vi "Actor Core.vi"(8 "error in":errorcluster, 11 "Study Actor in":refnum<class "Study Actor.lvclass">) -> (0 "error out":errorcluster, 3 "Actor out":refnum<class "Actor.lvclass">)   [LabVIEW 2024, in "Study Actor.lvlib" / "Study Actor.lvclass"]
doc: "The user interface for this panel.\n\n----\nPlease see the following web address for additional documentation and tutorial information:\nhttp://www.mooregoodideas.com/mgi-panel-manager/\n\nAuthor: Derek Trepanier\n\nCopyright (c) 2018, Moore Good Ideas, Inc.\n\nAll rights reserved.\n\nRedistribution and use in source and binary forms, with or without modification, are permitted provided that the following conditions are met:\n\n * Redistributions of source code must retain the above copyright notice, this list of conditions and the following disclaimer.\n * Redistributions in binary form must reproduce the above copyright notice, this list of conditions and the following disclaimer in the documentation and/or other materials provided with the distribution.\n * Neither the name of Moore Good Ideas, Inc. nor the names of its contributors may be used to endorse or promote products derived from this software without specific prior written permission.\n\nTHIS SOFTWARE IS PROVIDED BY THE COPYRIGHT HOLDERS AND CONTRIBUTORS \"AS IS\" AND ANY EXPRESS OR IMPLIED WARRANTIES, INCLUDING, BUT NOT LIMITED TO, THE IMPLIED WARRANTIES OF MERCHANTABILITY AND FITNESS FOR A PARTICULAR PURPOSE ARE DISCLAIMED. IN NO EVENT SHALL THE COPYRIGHT OWNER OR CONTRIBUTORS BE LIABLE FOR ANY DIRECT, INDIRECT, INCIDENTAL, SPECIAL, EXEMPLARY, OR CONSEQUENTIAL DAMAGES (INCLUDING, BUT NOT LIMITED TO, PROCUREMENT OF SUBSTITUTE GOODS OR SERVICES; LOSS OF USE, DATA, OR PROFITS; OR BUSINESS INTERRUPTION) HOWEVER CAUSED AND ON ANY THEORY OF LIABILITY, WHETHER IN CONTRACT, STRICT LIABILITY, OR TORT (INCLUDING NEGLIGENCE OR OTHERWISE) ARISING IN ANY WAY OUT OF THE USE OF THIS SOFTWARE, EVEN IF ADVISED OF THE POSSIBILITY OF SUCH DAMAGE."
uses:
  Study Actor.lvclass
  C:/Program Files/National Instruments/LabVIEW 2024/vi.lib/MGI/Panel Manager/Panel Actor/Panel Actor/Panel Actor.lvclass
  <vilib>/ActorFramework/Actor/Actor.lvclass
  Study Actor.lvclass/Study Actor.ctl
  <vilib>/ActorFramework/Message Enqueuer/Message Enqueuer.lvclass/Message Enqueuer.ctl
  IStudy Actor Messages/Log Target Msg/Log Target Msg.lvclass/Log Target Msg.ctl
  <vilib>/ActorFramework/Message Enqueuer/Enqueue.vi
  <vilib>/ActorFramework/Stop Msg/Stop Msg.lvclass
  C:/Program Files/National Instruments/LabVIEW 2024/vi.lib/ActorFramework/Message/Message.lvclass
  Study Actor Messages/Stop Target Actor Msg/Stop Target Actor Msg.lvclass
  IStudy Actor Messages/Log Target Msg/Log Target Msg.lvclass
  <vilib>/Utility/LVClass/Get LV Class Name.vi
  <resource>/AFDebug/Generate Trace for Message.vi
  <vilib>/ActorFramework/Message Priority Queue/Priority Enqueue.vi
  <vilib>/MGI/Panel Manager/Panel Actor/Panel Actor/Panel Actor.lvclass
  C:/Program Files/National Instruments/LabVIEW 2024/vi.lib/ActorFramework/Actor/Actor.lvclass
  D:/git/HAL/MAL/Study/Study Actor/Study Actor/Study Actor.lvclass
  D:/git/HAL/MAL/Study/Study Actor/IStudy Actor/IStudy Actor.lvclass
  C:/Program Files/National Instruments/LabVIEW 2024/vi.lib/ni/Actors/Network Endpoint Actors/Nested Endpoint Caller/Nested Endpoint Caller/Nested Endpoint Caller.lvclass
panel:
  in  "Launch Target":bool
  in  "Kill Target Button":bool
  out "Target Log":string
  out "Target Connected":bool
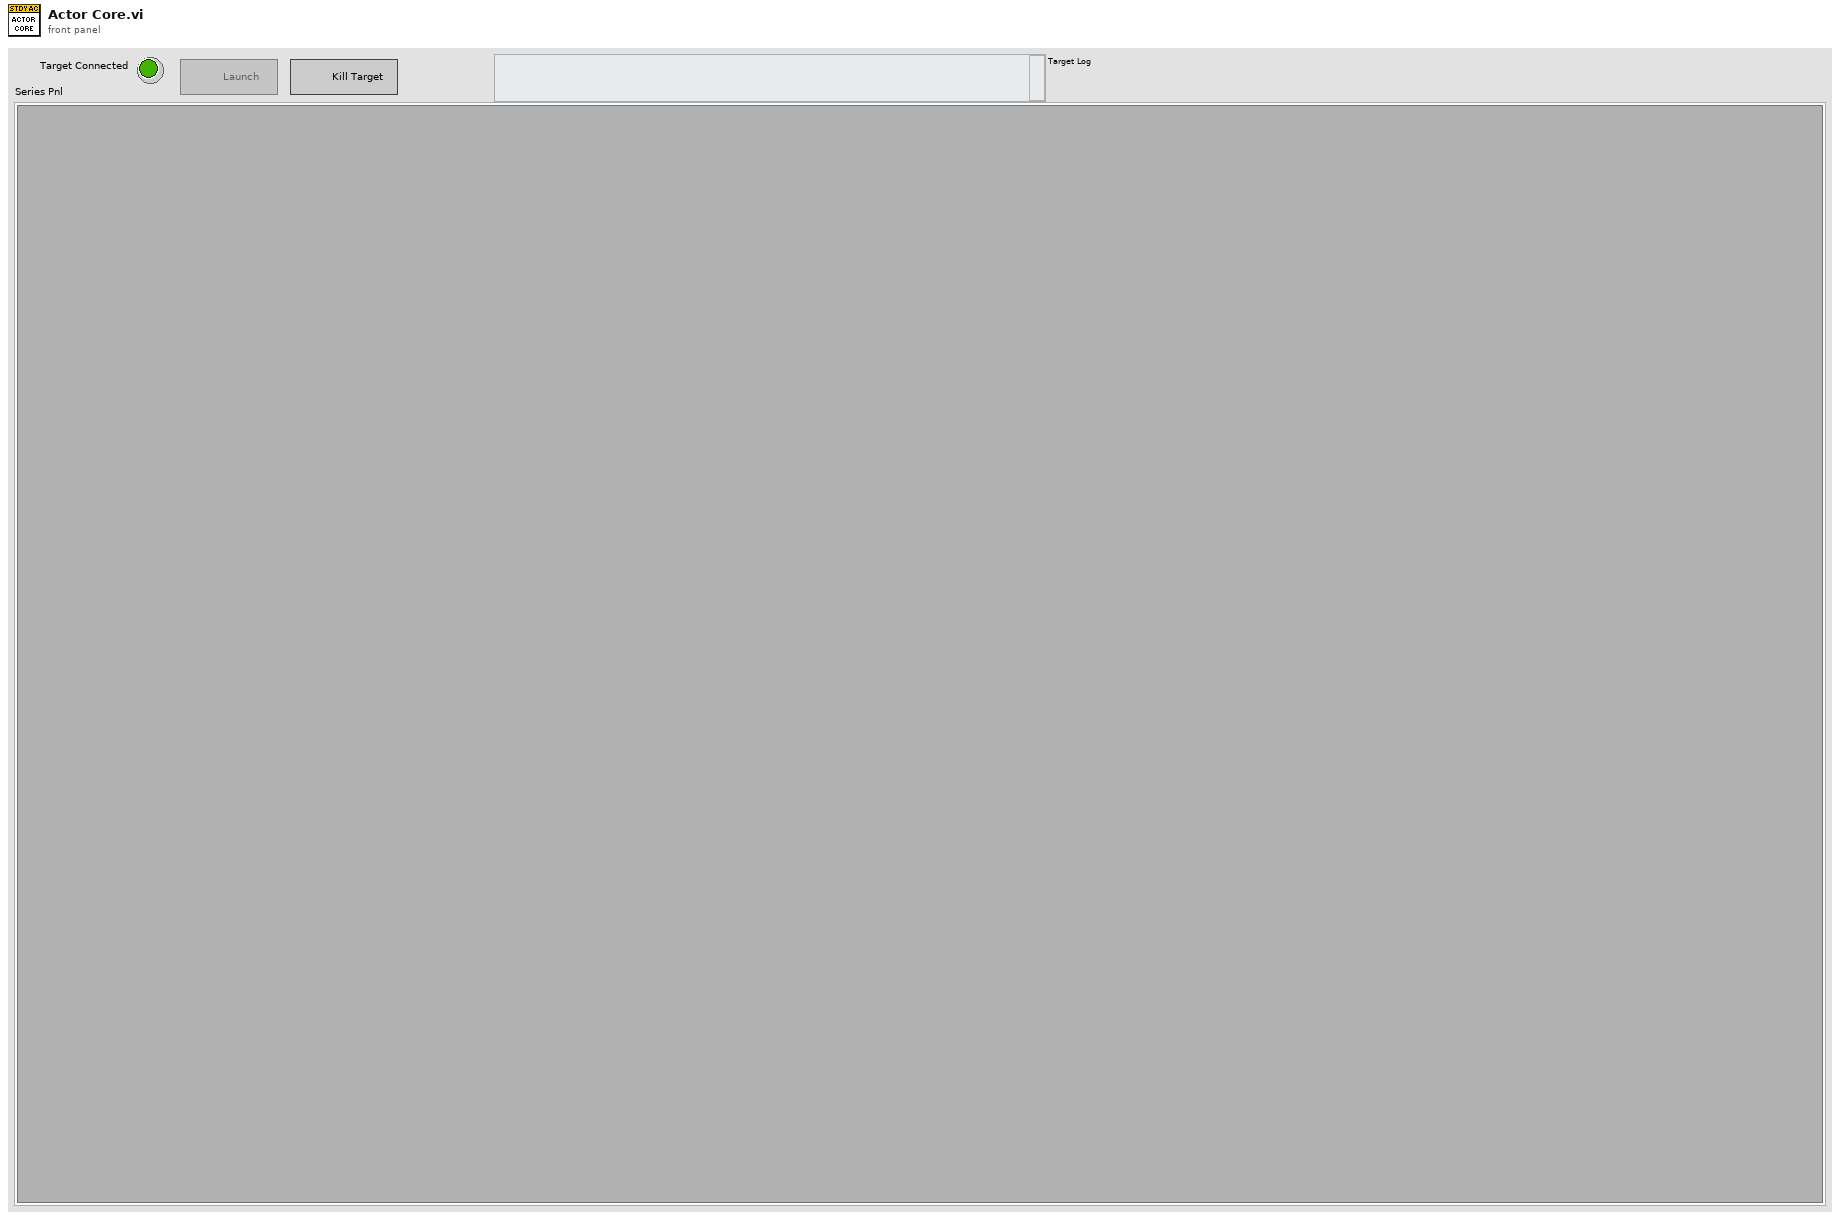
[diagram p1: front panel]
types:
  T1 = cluster{"Connected":refnum<user-event>, "Target Log Entry":refnum<user-event>}
  T2 = cluster{"Pnl Actor":refnum<event-registration>, "Event Registration Refnum":refnum<event-registration>}
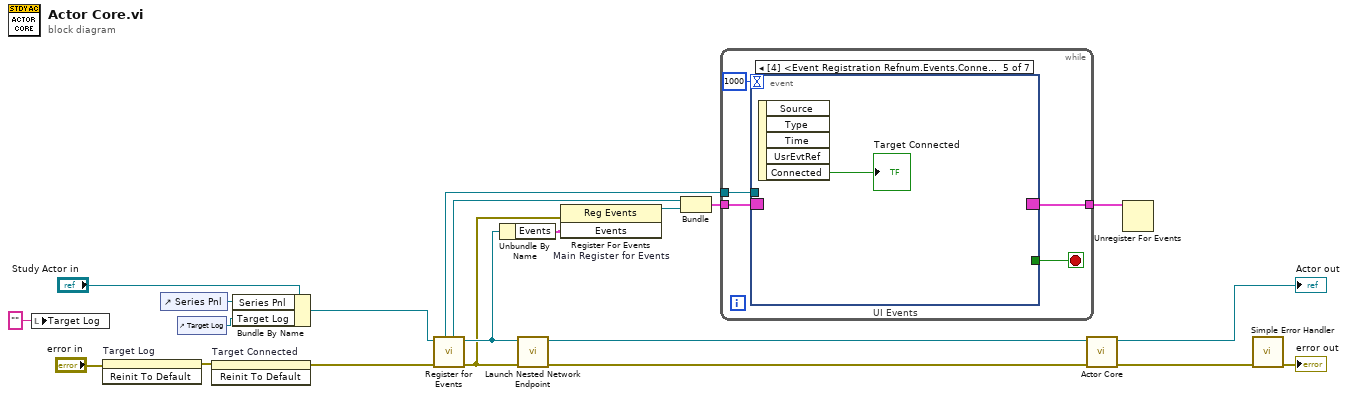
[diagram p0: block diagram]
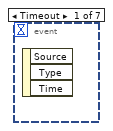
[diagram p2: hidden frame]
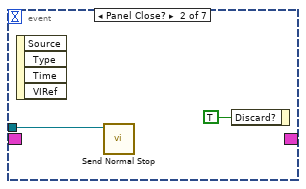
[diagram p3: hidden frame]
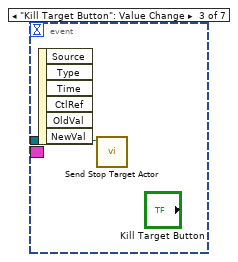
[diagram p4: hidden frame]
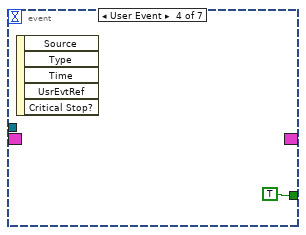
[diagram p5: hidden frame]
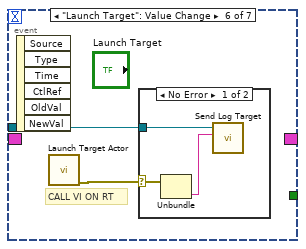
[diagram p6: hidden frame]
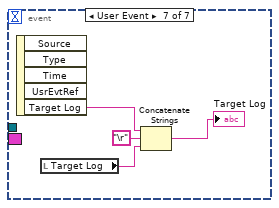
[diagram p8: hidden frame]
diagram:
  n1 = local write "Target Log"("") -> ()
  n2 = invoke on="Target Log" class="Str" method="Reinit To Default"(error in="error in") -> (error out=w5:errorcluster)  [unwired: 2 in, 2 out]
  n3 = control-ref of="Series Pnl"() -> (w18:refnum<vi>)
  n4 = control-ref of="Target Log"() -> (w7:refnum<vi>)
  n5 = invoke on="Target Connected" class="Bool (strict)" method="Reinit To Default"(error in=w5) -> (error out=w4:errorcluster)  [unwired: 2 in, 2 out]
  n6 = Bundle By Name(cluster="Study Actor in", "Series Pnl"=w18, "Target Log"=w7) -> (w17:refnum<class "Study Actor.lvclass">)
  n7 = call <vilib>:"Register for Events.vi"("Error In"=w4, "Panel Actor in"=w17) -> ("Error Out"=w8:errorcluster, "Panel Actor out"=w9:refnum<class "Study Actor.lvclass">, "Pnl Actor"=w13:refnum<event-registration>, "Self Enqueuer"=w12:refnum<class "Message Enqueuer.lvclass">)  [unwired: 6 in]
  n8 = Unbundle By Name(w9) -> ("Events"=w14:T1)
  n9 = call "Launch Nested Network Endpoint.vi"("error in"=w8, "Study Actor in"=w9) -> ("error out"=w11:errorcluster, "Study Actor out"=w10:refnum<class "Study Actor.lvclass">)  [unwired: 8 in]
  n10 = register-events "Main Register for Events"(error in=w8, w14) -> (reference out=w16:refnum<event-registration>)  [unwired: 1 in, 1 out]
  n11 = Bundle("Pnl Actor"=w13, "Event Registration Refnum"=w16) -> (w15:T2)  [unwired: 1 in]
  n12 = while {
    tunnel: w15 -> [w26]
    tunnel: w12 -> [w25]
    tunnel: [w22] -> w2
    stop <- w23 stop-if-true
    n13 = event "UI Events" shown="[4] <Event Registration Refnum.Events.Connected>: User Event" {
      selector: w26 -> [_ _ _ _ _ _ _]
      dyn-events: [_ _ _ _ _ _ _] -> w22
      timeout: 1000 -> [_ _ _ _ _ _ _]
      tunnel: [_ _ _ TRUE _ _ _] -> w23
      tunnel: w25 -> [_ w28 w29 _ _ w32 _]
      event Timeout {
        n14 = event-data() -> ()  [unwired: 1 in, 3 out]
      }
      event Panel Close? {
        n15 = event-data() -> ()  [unwired: 1 in, 4 out]
        n16 = call <vilib>:"Send Normal Stop.vi"("Message Enqueuer"=w28) -> ()  [unwired: 10 in, 1 out]
        n17 = event-data("Discard?"=TRUE) -> ()  [unwired: 1 in, 1 out]
      }
      event "Kill Target Button": Value Change {
        n18 = event-data() -> ()  [unwired: 1 in, 6 out]
        n19 = call "Send Stop Target Actor.vi"("Message Enqueuer"=w29) -> ()  [unwired: 9 in, 2 out]
      }
      event User Event {
        n20 = event-data() -> ()  [unwired: 1 in, 5 out]
      }
      event User Event {
        n21 = event-data() -> ("Connected"=→"Target Connected":bool)  [unwired: 1 in, 4 out]
      }
      event "Launch Target": Value Change {
        # "CALL VI ON RT"
        n22 = event-data() -> ()  [unwired: 1 in, 6 out]
        n23 = call "Launch Target Actor.vi"() -> ("error out"=w33:errorcluster)  [unwired: 11 in]
        n24 = case shown="No Error" w33 {
          selector: w33 -> [w35 _]
          tunnel: w32 -> [w36 _]
          frame No Error {
            n25 = Unbundle(w35) -> ("source"=w34:string)  [unwired: 2 out]
            n26 = call "Send Log Target.vi"("Entry"=w34, "Message Enqueuer"=w36) -> ()  [unwired: 8 in, 2 out]
          }
          frame Error {
          }
        }
      }
      event User Event {
        n27 = event-data() -> ("Target Log"=w40:string)  [unwired: 1 in, 4 out]
        n28 = local read "Target Log"() -> (w38:string)
        n29 = Concatenate Strings(w40, "\r", w38) -> (→"Target Log":string)
      }
    }
  }
  n30 = call-parent "Actor Core.vi"("error in"=w11, "Panel Actor in"=w10) -> ("error out"=w21:errorcluster, "Actor out"=→"Actor out":refnum<class "Actor.lvclass">)  [unwired: 8 in]
  n31 = Unregister For Events(event registration refnum=w2) -> ()  [unwired: 1 in, 1 out]
  n32 = call <vilib>:"Simple Error Handler.vi"("error in (no error)"=w21) -> ("error out"=→"error out":errorcluster)  [unwired: 4 in, 4 out]
